vi "spectrum.vi"(10 "z in":dbl[][](array[numeric]), 11 "Momentum [MeV/C]":dbl[](array[numeric])) -> (1 "output cluster":cluster{"dp [MeV/C]":dbl[], dbl[]}(graph))   [LabVIEW 2011]
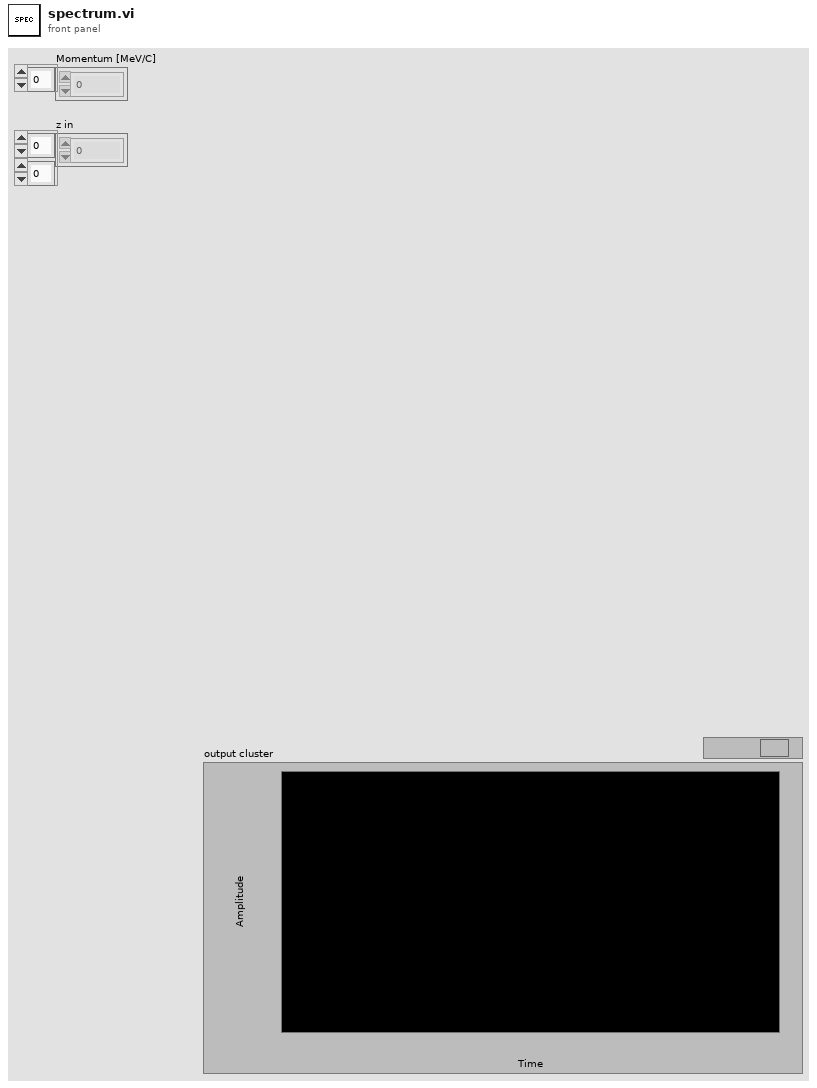
[diagram p1: front panel]
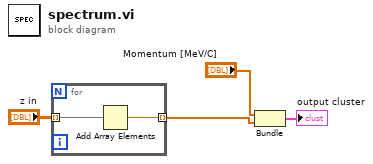
[diagram p0: block diagram]
diagram:
  n1 = for {
    tunnel: "z in" -> [w6] mode=indexing
    tunnel: [w5] -> w1 mode=indexing
    n2 = Add Array Elements(numeric array=w6) -> (sum=w5:dbl)
  }
  n3 = Bundle("Momentum [MeV/C]"="Momentum [MeV/C]", w1) -> (→"output cluster":cluster{"Momentum [MeV/C]":dbl[], dbl[]})  [unwired: 1 in]
